vi "AG-UC2-UC8_Open.vi"(6 "Instrument Key IN":string) -> (0 "error out":errorcluster, 1 "Error":i32, 2 "Instrument Key OUT":string, 3 "AG-UC2-UC8 Reference":refnum<k24>)   [LabVIEW 2020]
uses:
  C:/GEECS/Developers Version/builds/Device builds/AgilisPiezoStage/AgilisCmdLib.DLL
  AgilisCmdLib.DLL
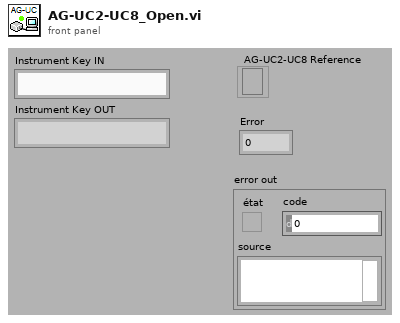
[diagram p1: front panel]
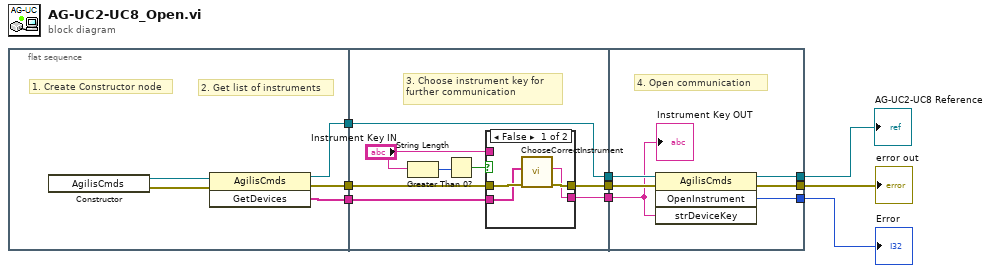
[diagram p0: block diagram]
diagram:
  n1 = flat-sequence {
    tunnel: [w12] -> w7
    tunnel: [w11] -> w6
    tunnel: [w10] -> w5
    tunnel: w7 -> [w17]
    tunnel: w6 -> [w19]
    tunnel: w5 -> [w18]
    tunnel: [w17] -> w4
    tunnel: [w16] -> w3
    tunnel: [w15] -> w2
    tunnel: [w34] -> w9
    tunnel: [w33] -> w8
    tunnel: w4 -> [w32]
    tunnel: w3 -> [w31]
    tunnel: w2 -> [w30]
    tunnel: [w29] -> w1
    frame #0 {
      # "2. Get list of instruments"
      # "1. Create Constructor node"
      n2 = constructor class="AgilisCmds"() -> (reference out=w14:refnum<k24>, error out=w13:errorcluster)  [unwired: 3 in, 1 out]
      n3 = invoke class="AgilisCmds" method="GetDevices"(reference=w14, error in=w13) -> (reference out=w12:refnum<k24>, error out=w11:errorcluster, "GetDevices"=w10:string[])  [unwired: 1 in]
    }
    frame #1 {
      # "3. Choose instrument key for \nfurther communication"
      n4 = String Length(string="Instrument Key IN") -> (length=w20:i32)
      n5 = Greater Than 0?(x=w20) -> (x > 0?=w21:bool)
      n6 = case shown="False" w21 {
        tunnel: w19 -> [w26 w28]
        tunnel: [w25 w28] -> w16
        tunnel: [w24 w27] -> w15
        tunnel: "Instrument Key IN" -> [_ w27]
        tunnel: w18 -> [w23 _]
        frame False {
          n7 = call "ChooseCorrectInstrument.vi"("Instrument Keys"=w23, "error in (no error)"=w26) -> ("Selected Instrument Key"=w24:string, "error out"=w25:errorcluster)  [unwired: 7 in]
        }
        frame True {
        }
      }
    }
    frame #2 {
      # "4. Open communication"
      n8 = invoke class="AgilisCmds" method="OpenInstrument"(reference=w32, error in=w31, "strDeviceKey"=w30) -> (reference out=w34:refnum<k24>, error out=w33:errorcluster, "OpenInstrument"=w29:i32)  [unwired: 1 in, 1 out]
      "Instrument Key OUT" <- w30
    }
  }
  "error out" <- w8
  "Error" <- w1
  "AG-UC2-UC8 Reference" <- w9
